vi "190627_AFTO.vi"() -> ()   [LabVIEW 2019]
uses:
  <vilib>/rvi/interface/nirviReadWriteControl/nirviReadWriteControl.xnode
  <vilib>/rvi/interface/Simulation/niFpgaSimulationCallBeginRW.vi
  <vilib>/rvi/errors/niLvFpgaAdjustHostInterfaceError.vi
  <vilib>/rvi/interface/nirviMethod/nirviMethod.xnode
  <vilib>/FPGAPlugInAG/Dynamic/niLvFpga_Reset_Dynamic.vi
  <vilib>/FPGAPlugInAG/Dynamic/niLvFpga_Run_Dynamic.vi
  <vilib>/rvi/interface/nirviCloseFPGA/nirviCloseFPGA.xnode
  <vilib>/Platform/TimedLoop/XDataNode/XDataNode.xnode
  <vilib>/Platform/TimedLoop/XDataNode/nitl_modes.ctl
  <vilib>/Platform/TimedLoop/XDataNode/XDNodeRunTimeDep.lvlib
  <vilib>/Platform/TimedLoop/XDataNode/wakeup.ctl
  <vilib>/Platform/TimedLoop/XDataNode/timing_clust.ctl
  <vilib>/rvi/interface/nirviOpenFPGA/nirviOpenFPGA.xnode
  <vilib>/Utility/Variable/NI_VariableUtilities.lvlib
  FPGA_TwoAxisEncoder_revised.vi
  <vilib>/FPGAPlugInAG/Dynamic/niLvFpga_Close_Dynamic.vi
panel:
  in  "Z_eta":dbl=-50.0 format="%#_13g"
  in  "X_eta":dbl=-50.0 format="%#_13g"
  out "LMS":bool
  in  "X_Type":string(combo)="Notch15"
  in  "Z_Type":string(combo)="Notch15"
  out "Time Slots (sec)":dbl[](array[numeric])
  out "All times (sec)":dbl
  out "one period  length":i32
  out "one period start time":i32
  in  "HOST Sample Rate (Hz)":i32=1000
  in  "LOAD":bool
  out "(LS) RMS X (one) (um)":dbl format="%0.4f"
  out "(LS) MAX ERROR X (um)":dbl format="%0.4f"
  out "(LS) RMS ERROR X (um)":dbl format="%0.4f"
  out "(En) RMS X (one) (um)":dbl format="%0.4f"
  out "(LS) RMS Z (one) (um)":dbl format="%0.4f"
  out "(LS) MAX ERROR Z (um)":dbl format="%0.4f"
  out "(LS) RMS ERROR Z (um)":dbl format="%0.4f"
  out "CMD X (rpm)":dbl[](graph)
  out "Linear Scale Position X (mm)":dbl[](graph)
  out "Linear Scale Position Z (mm)":dbl[](graph)
  out "(En) RMS Z (one) (um)":dbl format="%0.4f"
  out "CMD Z (rpm)":dbl[](graph)
  out "Position X (mm)":dbl[](graph)
  out "Linear Scale Position Error X (um)":dbl[](graph)
  out "Linear Scale Position Error Z (um)":dbl[](graph)
  out "Delay":i32
  out "(En) MAX ERROR X (um)":dbl format="%0.4f"
  out "(En) RMS ERROR X (um)":dbl format="%0.4f"
  out "Encoder Position Error X (um)":dbl[](graph)
  out "Position Command X (mm)":dbl[](graph)
  out "(En) MAX ERROR Z (um)":dbl format="%0.4f"
  out "(En) RMS ERROR Z (um)":dbl format="%0.4f"
  out "Encoder Position Error Z (um)":dbl[](graph)
  in  "RUN":bool
  in  "CLEAR":bool
  out "V Loop":bool
  out "Length(Response)":i32
  out "Length(Command)":i32
  out "Done":bool
  out "Error Out (FPGA)":errorcluster
  out "Error Out (Host)":errorcluster
  out "Position Z (mm)":dbl[](graph)
  out "FPGA INITIALIZED":bool
  in  "FPGA Sample Rate (Hz)":dbl=100000.0
  out "Position Command Z (mm)":dbl[](graph)
  in  "STOP":bool
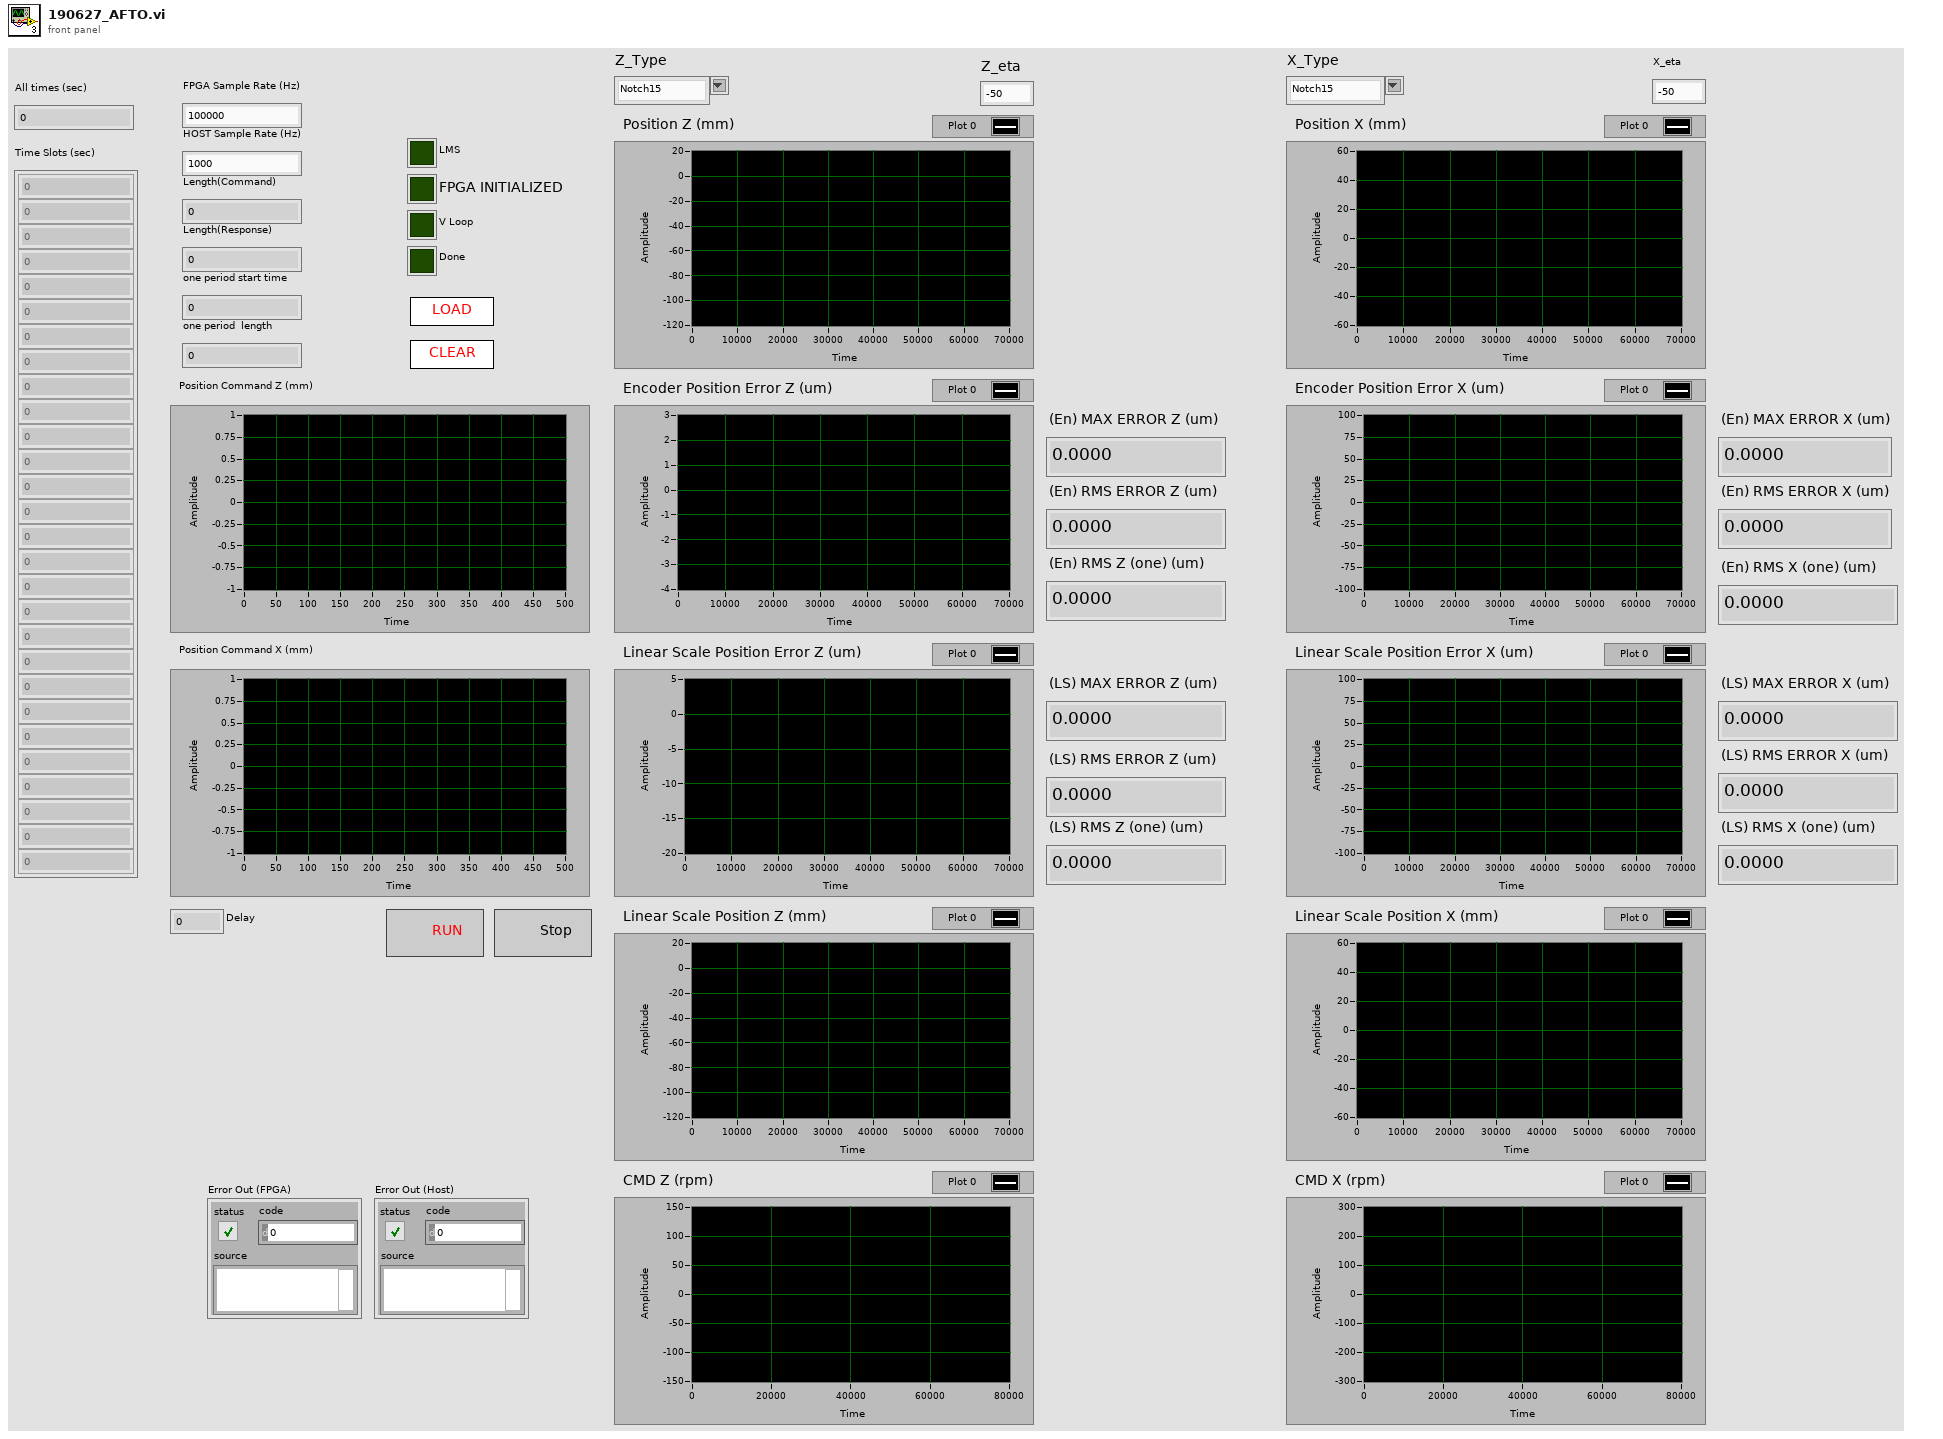
[diagram p1: front panel]
types:
  T1 = typedef "XDNodeRunTimeDep.lvlib/timing_clust.ctl" = cluster{"Expected End [f-1]":u64, "Actual End [f-1]":u64, "Finished Late? [f-1]":bool, "Expected End [i-1]":u64, "Actual End [i-1]":u64, "Finished Late? [i-1]":bool, "Expected Start [i]":u64, "Actual Start [i]":u64, "Expected Start [f]":u64, "Actual Start [f]":u64, "Source Name":string, "Structure Name":string, "Period":i64, "Deadline":i64, "Offset":i64, "Start":i64, "Priority":i32, "Timeout":i32, "Mode":T2, "Wakeup Reason":T3, "Error":errorcluster, "Source Type":string, "Secondary Source Type":string, "Global End Time":u64, "Global Start Time":u64, "Frame Duration":u64, "Iteration Duration":u64, "Assigned CPU":i32, "I/O Scan Engine Mode":u32}
  T2 = typedef "XDNodeRunTimeDep.lvlib/nitl_modes.ctl" = enum32{"No Change", "Process missed periods, maintain original phase", "Discard missed periods, maintain original phase", "Process missed periods, ignore original phase", "Discard missed periods, ignore original phase"}
  T3 = typedef "XDNodeRunTimeDep.lvlib/wakeup.ctl" = enum32{"Normal", "Aborted", "Asynchronous wakeup", "Timing source error", "Timed loop error", "Timeout"}
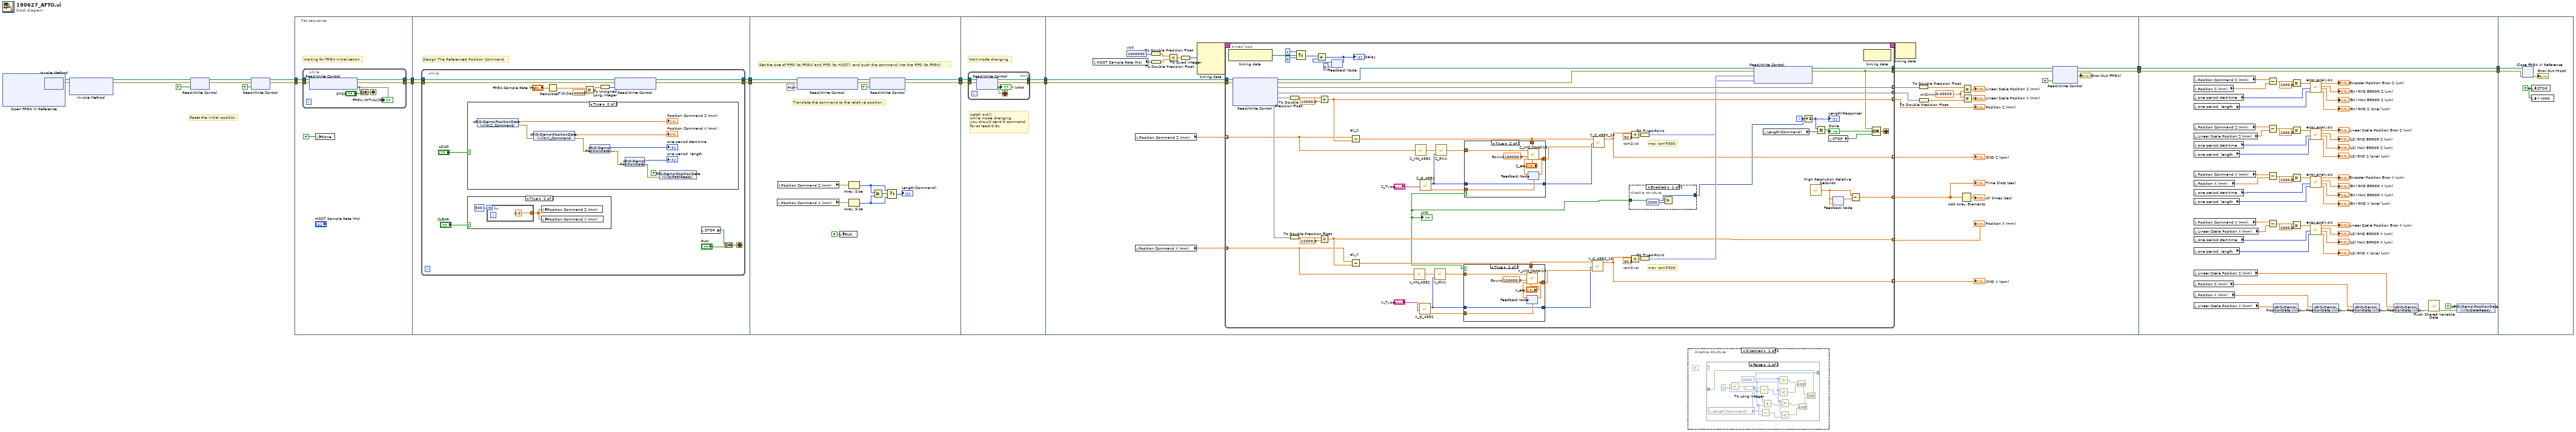
[diagram p0: block diagram]
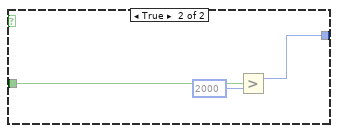
[diagram p2: hidden frame]
diagram:
  # "Reset the initial position"
  n1 = xnode "Open FPGA VI Reference"() -> ("FPGA VI Reference Out"=w7:refnum<k20>, "error out"=w6:errorcluster)  [unwired: 2 in]
  n2 = xnode "Invoke Method"("FPGA VI Reference In"=w7, "error in"=w6) -> ("FPGA VI Reference Out"=w20:refnum<k20>, "error out"=w19:errorcluster)
  n3 = xnode "Invoke Method"("FPGA VI Reference In"=w20, "error in"=w19) -> ("FPGA VI Reference Out"=w5:refnum<k20>, "error out"=w4:errorcluster)  [unwired: 1 in]
  n4 = xnode "Read/Write Control"("FPGA VI Reference In"=w5, "error in"=w4, "Initial"=TRUE ("Reset Encoder")) -> ("FPGA VI Reference Out"=w3:refnum<k20>, "error out"=w2:errorcluster)
  n5 = xnode "Read/Write Control"("FPGA VI Reference In"=w3, "error in"=w2, "Start"=TRUE) -> ("FPGA VI Reference Out"=w14:refnum<k20>, "error out"=w13:errorcluster)
  n6 = flat-sequence {
    tunnel: w14 -> [w29]
    tunnel: w13 -> [w28]
    tunnel: [w27] -> w24
    tunnel: [w26] -> w23
    tunnel: w24 -> [w40]
    tunnel: w23 -> [w39]
    tunnel: [w38] -> w22
    tunnel: [w37] -> w21
    tunnel: w22 -> [w76]
    tunnel: [w79] -> w18
    tunnel: w21 -> [w75]
    tunnel: [w78] -> w16
    tunnel: w18 -> [w83]
    tunnel: [w81] -> w17
    tunnel: w16 -> [w82]
    tunnel: [w80] -> w15
    tunnel: w17 -> [w119]
    tunnel: [w116] -> w11
    tunnel: w15 -> [w118]
    tunnel: [w109] -> w8
    tunnel: w11 -> [w264]
    tunnel: [w264] -> w10
    tunnel: [w263] -> w9
    tunnel: w8 -> [w263]
    tunnel: w10 -> [w267]
    tunnel: w9 -> [w266]
    frame #0 {
      # "Waiting for FPGA Initialization"
      n7 = while {
        tunnel: w29 -> [w36]
        tunnel: w28 -> [w33]
        tunnel: [w32] -> w26
        tunnel: [w31] -> w27
        stop <- w35 stop-if-true
        n8 = xnode "Read/Write Control"("FPGA VI Reference In"=w36, "error in"=w33) -> ("FPGA VI Reference Out"=w31:refnum<k20>, "error out"=w32:errorcluster, "SYSTEM INITIALIZED"=w30)
        "FPGA INITIALIZED" <- w30
        n9 = Or(x=w30, y="STOP") -> (x .or. y?=w35:bool)
      }
      n10 = local write "Done"(FALSE ("Done")) -> ()
    }
    frame #1 {
      # "Design The Referenced Position Command"
      n11 = while {
        tunnel: w40 -> [w54]
        tunnel: w39 -> [w53]
        tunnel: [w48] -> w38
        tunnel: [w47] -> w37
        stop <- w46 stop-if-true
        w50 = 40000000.0  # Tick/Sec
        n12 = case shown="True" "LOAD" {
          frame False {
          }
          frame True {
            n13 = shared-variable "cRIO-Demo\\PositionData.lvlib\\Z_Command"() -> (→"Position Command Z (mm)":dbl[], error out=w65:errorcluster)  [unwired: 1 in]
            n14 = shared-variable "cRIO-Demo\\PositionData.lvlib\\X_Command"(error in=w65) -> (→"Position Command X (mm)":dbl[], error out=w61:errorcluster)
            n15 = shared-variable "cRIO-Demo\\PositionData.lvlib\\t0"(error in=w61) -> (→"one period start time":i32, error out=w62:errorcluster)
            n16 = shared-variable "cRIO-Demo\\PositionData.lvlib\\tL"(error in=w62) -> (→"one period  length":i32, error out=w60:errorcluster)
            n17 = shared-variable "cRIO-Demo\\PositionData.lvlib\\PathReady"(FALSE ("PathReady"), error in=w60) -> ()  [unwired: 1 out]
          }
        }
        n18 = case shown="True" "CLEAR" {
          frame False {
          }
          frame True {
            n19 = for {
              N: 500 -> [_]
              tunnel: [0.0 ("element")] -> w56 mode=indexing
            }
            n20 = local write "Position Command Z (mm)"(w56) -> ()
            n21 = local write "Position Command X (mm)"(w56) -> ()
          }
        }
        n22 = Reciprocal(x="FPGA Sample Rate (Hz)") -> (1/x=w51:dbl)
        n23 = Multiply(x=w51, y=w50) -> (x*y=w52:dbl)
        n24 = To Unsigned Long Integer(number=w52) -> (unsigned 32bit integer=w49:u32)
        n25 = xnode "Read/Write Control"("FPGA VI Reference In"=w54, "error in"=w53, "Loop Delay (Tick)"=w49) -> ("FPGA VI Reference Out"=w48:refnum<k20>, "error out"=w47:errorcluster)
        n26 = local read "STOP"() -> (w45:bool)
        n27 = Or(x=w45, y="RUN") -> (x .or. y?=w46:bool)
      }
    }
    frame #2 {
      # "Translate the command to the relative position"
      # "Set the size of FIFO (to FPGA) and FIFO (to HOST), and push the command into the FIFO (to FPGA)"
      n28 = local read "Position Command X (mm)"() -> (w67:dbl[])
      n29 = local read "Position Command Z (mm)"() -> (w68:dbl[])
      n30 = xnode "Read/Write Control"("FPGA VI Reference In"=w76, "Output Votage Bound (vol)"=fxp<+,20,5> 10.0) -> ()  [unwired: 1 in, 2 out]
      n31 = local write "RUN"(FALSE) -> ()
      n32 = Array Size(array=w68) -> (size(s)=w71:i32)
      n33 = Array Size(array=w67) -> (size(s)=w70:i32)
      n34 = xnode "Read/Write Control"("FPGA VI Reference In"=w76, "error in"=w75, "HOST READY?"=TRUE) -> ("FPGA VI Reference Out"=w79:refnum<k20>, "error out"=w78:errorcluster)
      n35 = Greater Or Equal?(x=w71, y=w70) -> (x >= y?=w72:bool)
      n36 = Select(t=w71, s=w72, f=w70) -> (s? t:f=→"Length(Command)":i32)
    }
    frame #3 {
      # "watch out!!!\nwhile mode changing\nyou should send 0 command\nfor at least 0.5s."
      # "Wait mode changing"
      n37 = while {
        tunnel: w83 -> [w88]
        tunnel: w82 -> [w87]
        tunnel: [w86] -> w81
        tunnel: [w85] -> w80
        stop <- w84 stop-if-true
        n38 = xnode "Read/Write Control"("FPGA VI Reference In"=w88, "error in"=w87) -> ("FPGA VI Reference Out"=w86:refnum<k20>, "error out"=w85:errorcluster, "V Loop"=w84)
        "V Loop" <- w84
      }
    }
    frame #4 {
      w91 = 0.00025  # cnt2mm
      w113 = 1000000  # us/s
      n39 = local read "HOST Sample Rate (Hz)"() -> (w102:i32)
      n40 = local read "Position Command X (mm)"() -> (w100:dbl[])
      n41 = local read "Position Command Z (mm)"() -> (w101:dbl[])
      n42 = To Double Precision Float(number=w113) -> (double precision float=w105:dbl)
      n43 = To Double Precision Float(number=w102) -> (double precision float=w106:dbl)
      n44 = Divide(x=w105, y=w106) -> (x/y=w112:dbl)
      n45 = To Quad Integer(1:w112) -> (0:w111:i64)
      n46 = node-c288(w111) -> (w115:T1)  [unwired: 3 in]
      n47 = timed-loop {
        tunnel: w119 -> [w163]
        tunnel: w118 -> [w161]
        tunnel: [w147] -> w117
        timing: w115 -> [_]
        timing-out: [_] -> w114
        tunnel: [w146] -> w110
        tunnel: [w157] -> w96 mode=indexing
        tunnel: [w154] -> w94 mode=indexing
        tunnel: [w135] -> w103 mode=indexing
        tunnel: [w158] -> w95 mode=indexing
        tunnel: w101 -> [w133] mode=indexing
        tunnel: w100 -> [w129] mode=indexing
        tunnel: [w122] -> w99 mode=indexing
        tunnel: [w152] -> w93 mode=indexing
        tunnel: [w142] -> w89 mode=indexing
        i -> [w121]
        stop <- w178 stop-if-true
        w156 = 30.0  # rpm2vol
        w174 = 30.0  # rpm2vol
        # "max rpm=300"
        # "max rpm=300"
        n48 = node-c288() -> (w168:bool)  [unwired: 1 in]
        n49 = xnode "Read/Write Control"("FPGA VI Reference In"=w163, "error in"=w161) -> ("FPGA VI Reference Out"=w151:refnum<k20>, "error out"=w150:errorcluster, "Line Scale Z (count)"=w154, "Line Scale X (count)"=w152, "Encoder Z (count)"=w153, "Encoder X (count)"=w145)
        n50 = To Double Precision Float(number=w153) -> (double precision float=w173:dbl)
        n51 = To Double Precision Float(number=w145) -> (double precision float=w160:dbl)
        n52 = Select(t=1, s=w168, f=0) -> (s? t:f=w167:i32)
        n53 = Divide(x=w173, y=10000.0) -> (x/y=w157:dbl)
        n54 = Divide(x=w160, y=12000.0) -> (x/y=w158:dbl)
        n55 = feedback #1(0) -> (w165:i32)
        n56 = Add(x=w167, y=w165) -> (x+y=w166:i32)
        "Delay" <- w166
        n57 = feedback-in #1(w166) -> ()
        n58 = Subtract "ek_Z"(x=w133, y=w157) -> (x-y=w134:dbl)
        n59 = Subtract "ek_X"(x=w129, y=w158) -> (x-y=w123:dbl)
        n60 = call "X_MN_4352.vi"("u"=w129) -> ("y"=w130:dbl)  [unwired: 4 in]
        n61 = call "Z_MN_4952.vi"("u"=w133) -> ("y"=w141:dbl)  [unwired: 4 in]
        n62 = call "X_Q_4352.vi"("Type"="X_Type") -> ("Qn"=w127:dbl[], "L"=w128:i32)  [unwired: 9 in]
        n63 = call "Z_Q_4952.vi"("Type"="Z_Type") -> ("Qn"=w138:dbl[], "L"=w139:i32)  [unwired: 9 in]
        n64 = call "X_Phik.vi"("Lq"=w128, "u"=w130) -> ("phik"=w131:dbl[])  [unwired: 3 in]
        n65 = call "Z_Phik.vi"("Lq"=w139, "u"=w141) -> ("phik"=w140:dbl[])  [unwired: 3 in]
        n66 = disable-structure shown="Enabled" {
          disable-tunnel: w121 -> [w180 _]
          disable-tunnel: [w179 _] -> w120
          frame Enabled {
            n67 = Greater?(x=w180, y=2000) -> (0:w179:bool)
          }
          frame Disabled {
          }
        }
        "LMS" <- w120
        n68 = case shown="True" w120 {
          tunnel: w123 -> [_ w191]
          tunnel: w131 -> [_ w190]
          tunnel: [w182 w186] -> w125
          tunnel: w127 -> [w182 w188]
          tunnel: w128 -> [w183 w187]
          tunnel: [w183 w187] -> w124
          frame False {
          }
          frame True {
            w185 = 100000.0  # Bound
            n69 = feedback #2(w188) -> (w189:dbl[])
            n70 = call "X_LMS_Notch15.vi"("eta"="X_eta", "ek"=w191, "q_input"=w189, "Bound"=w185, "phik"=w190) -> ("q_out"=w186:dbl[])  [unwired: 4 in]
            n71 = feedback-in #2(w186) -> ()
          }
        }
        n72 = case shown="True" w120 {
          tunnel: w134 -> [_ w201]
          tunnel: w140 -> [_ w200]
          tunnel: [w192 w195] -> w137
          tunnel: w138 -> [w192 w197]
          tunnel: w139 -> [w193 w196]
          tunnel: [w193 w196] -> w136
          frame False {
          }
          frame True {
            w194 = 100000.0  # Bound
            n73 = feedback #3(w197) -> (w198:dbl[])
            n74 = call "Z_LMS_Notch15.vi"("eta"="Z_eta", "ek"=w201, "q_input"=w198, "Bound"=w194, "phik"=w200) -> ("q_out"=w195:dbl[])  [unwired: 4 in]
            n75 = feedback-in #3(w195) -> ()
          }
        }
        n76 = call "X_C_4352_15.vi"("ek"=w123, "length"=w124, "q"=w125) -> ("uk"=w122:dbl)  [unwired: 4 in]
        n77 = call "Z_C_4952_15.vi"("ek"=w134, "length"=w136, "q"=w137) -> ("uk"=w135:dbl)  [unwired: 4 in]
        n78 = Divide(x=w135, y=w174) -> (x/y=w175:fxp<+/-,20,5>)
        n79 = Divide(x=w122, y=w156) -> (x/y=w155:fxp<+/-,20,5>)
        n80 = To Fixed-Point(number=w175) -> (fixed-point=w149:fxp<+/-,20,5>)  [unwired: 1 in]
        n81 = To Fixed-Point(number=w155) -> (fixed-point=w148:fxp<+/-,20,5>)  [unwired: 1 in]
        n82 = xnode "Read/Write Control"("FPGA VI Reference In"=w151, "error in"=w150, "Velocity Command Z (vol)"=w149, "Velocity Command X (vol)"=w148) -> ("FPGA VI Reference Out"=w147:refnum<k20>, "error out"=w146:errorcluster)
        n83 = local read "Length(Command)"() -> (w162:i32)
        n84 = Increment(x=w121) -> (x+1=w171:i32)
        "Length(Response)" <- w171
        n85 = call <vilib>:"High Resolution Relative Seconds.vi"() -> ("relative seconds"=w144:dbl)
        n86 = Greater Or Equal?(x=w171, y=w162) -> (x >= y?=w177:bool)
        "Done" <- w177
        n87 = local read "STOP"() -> (w176:bool)
        n88 = feedback #4(w144) -> (w143:dbl)
        n89 = feedback-in #4(w144) -> ()
        n90 = Subtract(x=w144, y=w143) -> (x-y=w142:dbl)
        n91 = node-c288() -> ()  [unwired: 1 in, 1 out]
        n92 = Compound Arithmetic op=OR(w146, w177, w176) -> (w178:bool)
      }
      "Position Z (mm)" <- w96
      "Position X (mm)" <- w95
      "CMD Z (rpm)" <- w103
      "CMD X (rpm)" <- w99
      "Time Slots (sec)" <- w89
      n93 = node-c288(w114) -> ()  [unwired: 1 out]
      n94 = To Double Precision Float(number=w94) -> (double precision float=w92:dbl[])
      n95 = To Double Precision Float(number=w93) -> (double precision float=w98:dbl[])
      n96 = Add Array Elements(numeric array=w89) -> (sum=→"All times (sec)":dbl)
      n97 = Multiply(x=w92, y=w91) -> (x*y=→"Linear Scale Position Z (mm)":dbl[])
      n98 = Multiply(x=w91, y=w98) -> (x*y=→"Linear Scale Position X (mm)":dbl[])
      n99 = xnode "Read/Write Control"("FPGA VI Reference In"=w117, "error in"=w110, "stop"=TRUE) -> ("FPGA VI Reference Out"=w116:refnum<k20>, "error out"=w109:errorcluster, "Error Out"=→"Error Out (FPGA)")
    }
    frame #5 {
      n100 = local read "Position Command Z (mm)"() -> (w262:dbl[])
      n101 = local read "Position Z (mm)"() -> (w261:dbl[])
      n102 = local read "one period start time"() -> (w252:i32)
      n103 = local read "one period  length"() -> (w251:i32)
      n104 = local read "Position Command Z (mm)"() -> (w215:dbl[])
      n105 = local read "Linear Scale Position Z (mm)"() -> (w258:dbl[])
      n106 = local read "one period start time"() -> (w246:i32)
      n107 = local read "one period  length"() -> (w245:i32)
      n108 = local read "Position Command X (mm)"() -> (w233:dbl[])
      n109 = local read "Position X (mm)"() -> (w232:dbl[])
      n110 = local read "one period start time"() -> (w231:i32)
      n111 = local read "one period  length"() -> (w230:i32)
      n112 = local read "Position Command X (mm)"() -> (w216:dbl[])
      n113 = local read "Linear Scale Position X (mm)"() -> (w229:dbl[])
      n114 = local read "one period start time"() -> (w228:i32)
      n115 = local read "one period  length"() -> (w227:i32)
      n116 = local read "Linear Scale Position Z (mm)"() -> (w225:dbl[])
      n117 = local read "Position Z (mm)"() -> (w217:dbl[])
      n118 = local read "Position X (mm)"() -> (w218:dbl[])
      n119 = local read "Linear Scale Position X (mm)"() -> (w226:dbl[])
      n120 = Subtract(x=w262, y=w261) -> (x-y=w259:dbl[])
      n121 = Subtract(x=w215, y=w258) -> (x-y=w210:dbl[])
      n122 = Subtract(x=w233, y=w232) -> (x-y=w243:dbl[])
      n123 = Subtract(x=w216, y=w229) -> (x-y=w214:dbl[])
      n124 = shared-variable "cRIO-Demo\\PositionData.lvlib\\X_LS"(w226) -> (error out=w224:errorcluster)  [unwired: 1 in]
      n125 = Multiply(x=w259, y=1000.0) -> (x*y=w257:dbl[])
      n126 = Multiply(x=w210, y=1000.0) -> (x*y=w209:dbl[])
      n127 = Multiply(x=w243, y=1000.0) -> (x*y=w244:dbl[])
      n128 = Multiply(x=w214, y=1000.0) -> (x*y=w212:dbl[])
      n129 = call "error_analysis.vi"("tLength"=w251, "t0"=w252, "data in (um)"=w257) -> ("rms (one) (um)"=→"(En) RMS Z (one) (um)":dbl, "max err (um)"=→"(En) MAX ERROR Z (um)":dbl, "rms (all) (um)"=→"(En) RMS ERROR Z (um)":dbl, "data out (um)"=→"Encoder Position Error Z (um)":dbl[])  [unwired: 5 in]
      n130 = call "error_analysis.vi"("tLength"=w245, "t0"=w246, "data in (um)"=w209) -> ("rms (one) (um)"=→"(LS) RMS Z (one) (um)":dbl, "max err (um)"=→"(LS) MAX ERROR Z (um)":dbl, "rms (all) (um)"=→"(LS) RMS ERROR Z (um)":dbl, "data out (um)"=→"Linear Scale Position Error Z (um)":dbl[])  [unwired: 5 in]
      n131 = call "error_analysis.vi"("tLength"=w230, "t0"=w231, "data in (um)"=w244) -> ("rms (one) (um)"=→"(En) RMS X (one) (um)":dbl, "max err (um)"=→"(En) MAX ERROR X (um)":dbl, "rms (all) (um)"=→"(En) RMS ERROR X (um)":dbl, "data out (um)"=→"Encoder Position Error X (um)":dbl[])  [unwired: 5 in]
      n132 = call "error_analysis.vi"("tLength"=w227, "t0"=w228, "data in (um)"=w212) -> ("rms (one) (um)"=→"(LS) RMS X (one) (um)":dbl, "max err (um)"=→"(LS) MAX ERROR X (um)":dbl, "rms (all) (um)"=→"(LS) RMS ERROR X (um)":dbl, "data out (um)"=→"Linear Scale Position Error X (um)":dbl[])  [unwired: 5 in]
      n133 = shared-variable "cRIO-Demo\\PositionData.lvlib\\X_EN"(w218, error in=w224) -> (error out=w223:errorcluster)
      n134 = shared-variable "cRIO-Demo\\PositionData.lvlib\\Z_EN"(w217, error in=w223) -> (error out=w222:errorcluster)
      n135 = shared-variable "cRIO-Demo\\PositionData.lvlib\\Z_LS"(w225, error in=w222) -> (error out=w221:errorcluster)
      n136 = call <vilib>:"Flush Shared Variable Data.vi"("error in (no error)"=w221) -> ("error out"=w220:errorcluster)  [unwired: 10 in]
      n137 = shared-variable "cRIO-Demo\\PositionData.lvlib\\DataReady"(TRUE, error in=w220) -> ()  [unwired: 1 out]
    }
    frame #6 {
      w265 = FALSE ("STOP")
      n138 = xnode "Close FPGA VI Reference"("FPGA VI Reference In"=w267, "error in"=w266) -> ("error out"=→"Error Out (Host)":errorcluster)
      n139 = local write "STOP"(w265) -> ()
      n140 = local write "V Loop"(w265) -> ()
    }
  }
  n141 = disable-structure shown="Disabled" {
    frame Disabled {
      w269 = FALSE
      n142 = case shown="False" {
        selector: _ -> [_ _]
        tunnel: _ -> [w278 w287]
        tunnel: [w273 w286] -> _
        frame False {
          w272 = 3500 ("y")
          n143 = local read "Length(Command)"() -> (w270:i32)
          n144 = Divide(x=w270, y=2) -> (x/y=w271:dbl)
          n145 = To Long Integer(number=w271) -> (32bit integer=w276:i32)
          n146 = Subtract(x=w276, y=w272) -> (x-y=w283:i32)
          n147 = Subtract(x=w270, y=w272) -> (x-y=w280:i32)
          n148 = Add(x=w276, y=w272) -> (x+y=w277:i32)
          n149 = Greater?(x=w278, y=w272) -> (0:w285:bool)
          n150 = Less?(x=w278, y=w283) -> (x < y?=w282:bool)
          n151 = Greater?(x=w278, y=w277) -> (0:w279:bool)
          n152 = Less?(x=w278, y=w280) -> (x < y?=w281:bool)
          n153 = And(x=w285, y=w282) -> (x .and. y?=w275:bool)
          n154 = And(x=w279, y=w281) -> (x .and. y?=w274:bool)
          n155 = Or(x=w275, y=w274) -> (x .or. y?=w273:bool)
        }
        frame True {
          n156 = Greater?(x=w287, y=2000) -> (0:w286:bool)
        }
      }
    }
    frame Enabled {
    }
  }
